vi "測試環境1.vi"() -> ()   [LabVIEW 2021]
panel:
  in  "輸入資料":dbl(slide) scale=0.0..100.0
  in  "停止":bool
  out "溫度計":dbl(xcontrol)
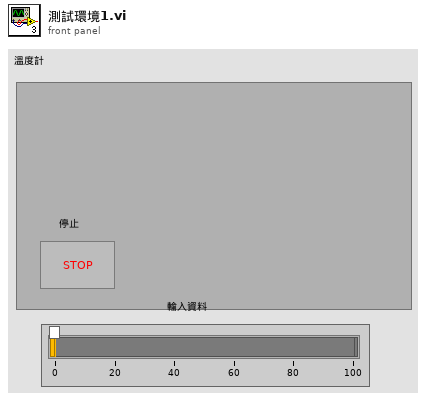
[diagram p1: front panel]
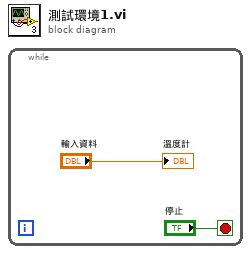
[diagram p0: block diagram]
diagram:
  n1 = while {
    stop <- "停止" stop-if-true
    "溫度計" <- "輸入資料"
  }
